vi "Remove_zeros.vi"(3 "subarray in":dbl[](array[numeric])) -> (1 "subarray out":dbl[](array[numeric]))   [LabVIEW 2016, in "CNN.lvclass"]
uses:
  biCNN/CNN.lvclass
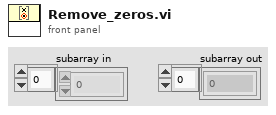
[diagram p1: front panel]
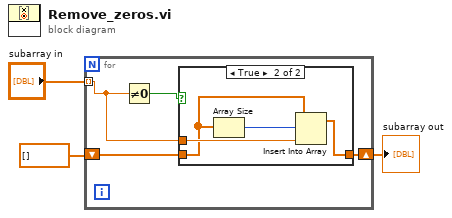
[diagram p0: block diagram]
diagram:
  n1 = for {
    tunnel: "subarray in" -> [w4] mode=indexing
    shift-right: [w5] -> w3
    shift-left: dbl[] [] ("subarray") -> [w6]
    n2 = Not Equal To 0?(x=w4) -> (x != 0?=w7:bool)
    n3 = case shown="True" w7 {
      tunnel: w6 -> [w8 w10]
      tunnel: [w8 w12] -> w5
      tunnel: w4 -> [_ w11]
      frame False {
      }
      frame True {
        n4 = Array Size(array=w10) -> (size(s)=w9:i32)
        n5 = Insert Into Array(array=w10, index=w9, new element=w11) -> (w12:dbl[])
      }
    }
  }
  "subarray out" <- w3
